vi "Filter.vi"(9 "FilterSpecification":refnum<class "IFilterSpecification.lvclass">, 10 "Products In":refnum<class "Product.lvclass">[](array[class]), 11 "BetterFilter":refnum<class "BetterFilter.lvclass">) -> (2 "Filtered Products":refnum<class "Product.lvclass">[](array[class]))   [LabVIEW 2018, in "BetterFilter.lvclass"]
uses:
  BetterFilter.lvclass
  IFilterSpecification/IFilterSpecification.lvclass
  Product/Product.lvclass
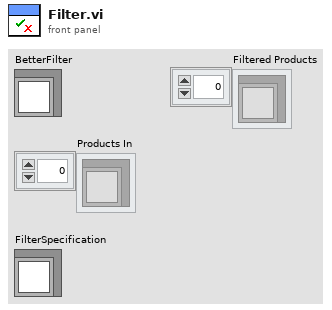
[diagram p1: front panel]
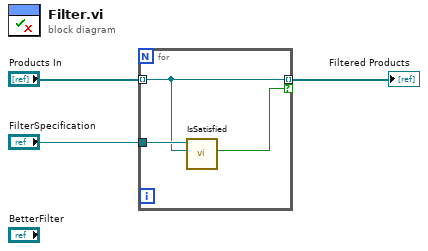
[diagram p0: block diagram]
diagram:
  n1 = for {
    tunnel: "Products In" -> [w5] mode=indexing
    tunnel: "FilterSpecification" -> [w6]
    tunnel: [w5] -> w1 mode=indexing if=w4
    n2 = call-dynamic "IsSatisfied.vi"("Product"=w5, "IFilterSpecification"=w6) -> ("IsSatisfied"=w4:bool)  [unwired: 9 in]
  }
  "Filtered Products" <- w1
